vi "Launch Common Measurements.vi"() -> ()   [LabVIEW 2015]
uses:
  Libraries/Mag Lab Measure/Common Measurements/Load App.vi
  Libraries/Mag Lab Measure/Common Measurements/Common Measurements.lvclass
panel:
  out "Waiting Lights":T1
  out "Current action:":string
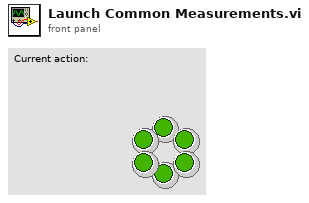
[diagram p1: front panel]
types:
  T1 = cluster{"DNL_wait 1":bool, "DNL_wait 1":bool, "DNL_wait 1":bool, "DNL_wait 1":bool, "DNL_wait 1":bool, "DNL_wait 1":bool}
  T2 = cluster{"[0]":bool, "[1]":bool, "[2]":bool, "[3]":bool, "[4]":bool, "[5]":bool}
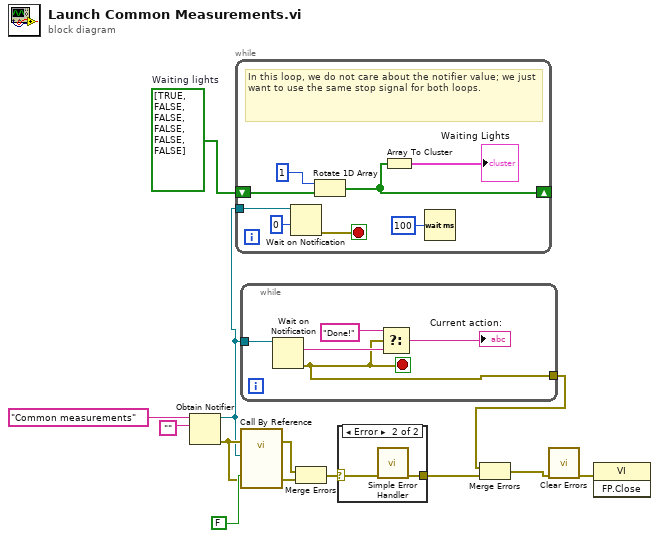
[diagram p0: block diagram]
diagram:
  w2 = bool[] [TRUE, FALSE, FALSE, FALSE, FALSE, FALSE]  # Waiting lights
  n1 = Obtain Notifier(name (unnamed)="Common measurements", notification data type="") -> (notifier out=w1:refnum<notifier>, error out=w8:errorcluster)  [unwired: 2 in, 1 out]
  n2 = while {
    shift-right: [w15] -> _
    shift-left: w2 -> [w17]
    tunnel: w1 -> [w19]
    stop <- w21 stop-if-true
    # "In this loop, we do not care about the notifier value; we just want to use the same stop signal for both loops."
    n3 = Wait on Notification(notifier=w19, timeout in ms (-1)=0) -> (error out=w21:errorcluster)  [unwired: 2 in, 3 out]
    n4 = Rotate 1D Array(1:w17, 2:1 ("n")) -> (0:w15:bool[])
    n5 = Array To Cluster(array=w15) -> (cluster=→"Waiting Lights":T2)
    n6 = Wait (ms)(milliseconds to wait=u32 100) -> ()  [unwired: 1 out]
  }
  n7 = while {
    tunnel: w1 -> [w26]
    tunnel: [w22] -> w3
    stop <- w22 stop-if-true
    n8 = Wait on Notification(notifier=w26) -> (notification=w24:string, error out=w22:errorcluster)  [unwired: 3 in, 2 out]
    n9 = Select(t="Done!" ("notification"), s=w22, f=w24) -> (s? t:f=→"Current action:":string)
  }
  n10 = call-by-ref "?"(error in=w8, "Open Actor Core front panel? (F)"=FALSE, "Error In"=w8, "Status Notifier"=w1) -> (error out=w11:errorcluster, "Error Out"=w7:errorcluster)  [unwired: 9 in, 1 out]
  n11 = Merge Errors(w11, w7) -> (w12:errorcluster)
  n12 = case shown="Error" w12 {
    selector: w12 -> [w27 w29]
    tunnel: [w27 w28] -> w5
    frame No Error {
    }
    frame Error {
      n13 = call <vilib>:"Simple Error Handler.vi"("error in (no error)"=w29) -> ("error out"=w28:errorcluster)  [unwired: 4 in, 4 out]
    }
  }
  n14 = Merge Errors(w3, w5) -> (w4:errorcluster)
  n15 = call <vilib>:"Clear Errors.vi"("error in (no error)"=w4) -> ("error out"=w13:errorcluster)  [unwired: 5 in, 1 out]
  n16 = invoke class="VI" method="FP.Close"(error in=w13) -> ()  [unwired: 2 in, 3 out]
